vi "Initialize CVT.vi"(8 "error in (no error)":errorcluster, 11 "Measurement in":refnum<class "Measurement.lvclass">) -> (0 "error out":errorcluster, 3 "Measurement out":refnum<class "Measurement.lvclass">)   [LabVIEW 2017, in "Measurement Actor.lvlib" / "Measurement.lvclass"]
uses:
  Measurement.lvclass
  Measurement.lvclass/Measurement.ctl
  <vilib>/NI/Current Value Table/Type Defs/File Format.ctl
  <vilib>/NI/Current Value Table/Type Defs/Single Tag.ctl
  <vilib>/NI/Current Value Table/Type Defs/Data Types.ctl
  <vilib>/NI/Current Value Table/Type Defs/Tag Grouping set.ctl
  <vilib>/NI/Current Value Table/Current Value Table.lvlib
  Hardware/Hardware.lvclass
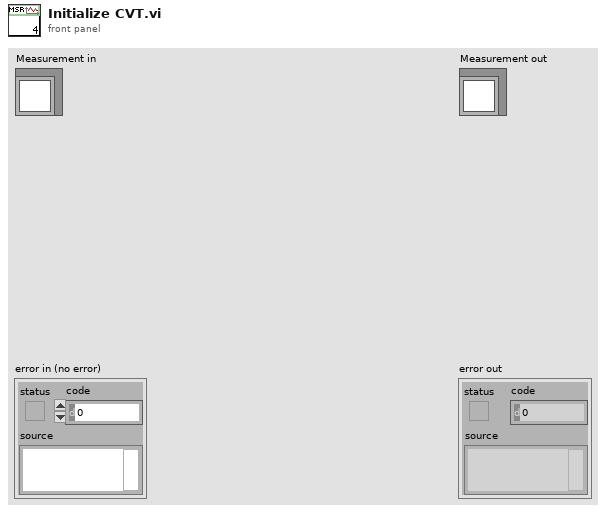
[diagram p1: front panel]
types:
  T1 = typedef "Current Value Table.lvlib/File Format.ctl" = cluster{"Tags":T2[], "Group Listings":T4[]}
  T2 = typedef "Current Value Table.lvlib/Single Tag.ctl" = cluster{"Data Type":T3, "Name":string, "Value":string, "Description":string}
  T3 = typedef "Current Value Table.lvlib/Data Types.ctl" = enum16{"Double", "Single", "I64", "I32", "I16", "I8", "U64", "U32", "U16", "U8", "String", "Boolean", "Array of U8", "Array of U16", "Array of U32", "Array of U64", "Array of I64", "Array of I32", "Array of I16", "Array of I8", "Array of Double", "Array of Single", "Array of Boolean", "Array of String"}
  T4 = typedef "Current Value Table.lvlib/Tag Grouping set.ctl" = cluster{"Group":string, "Tag Names":string[]}
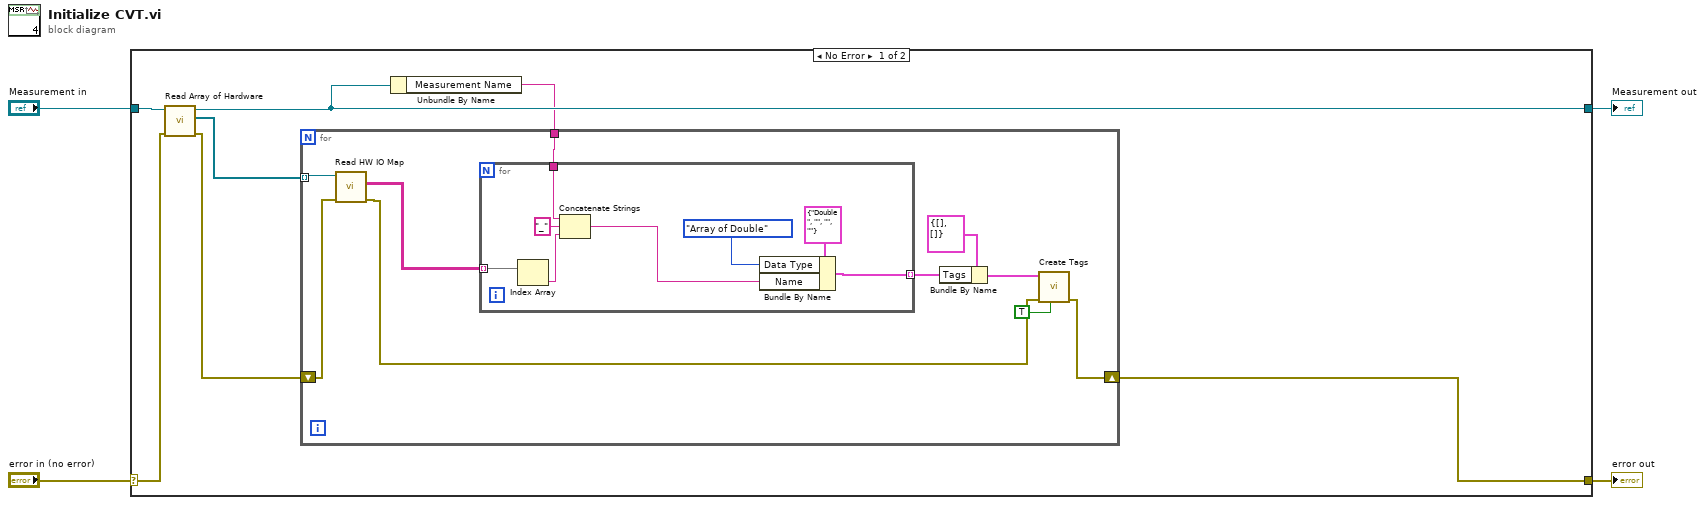
[diagram p0: block diagram]
diagram:
  n1 = case shown="No Error" "error in (no error)" {
    selector: "error in (no error)" -> [w6 w31]
    tunnel: [w5 w31] -> w3
    tunnel: [w9 w30] -> w1
    tunnel: "Measurement in" -> [w11 w30]
    frame No Error {
      n2 = call "Read Array of Hardware.vi"("error in (no error)"=w6, "Measurement in"=w11) -> ("error out"=w7:errorcluster, "Array of Hardware"=w10:refnum<class "Hardware.lvclass">[], "Measurement out"=w9:refnum<class "Measurement.lvclass">)  [unwired: 7 in]
      n3 = Unbundle By Name(w9) -> ("Measurement Name"=w8:string)
      n4 = for {
        tunnel: w10 -> [w16] mode=indexing
        tunnel: w8 -> [w18]
        shift-right: [w13] -> w5
        shift-left: w7 -> [w15]
        n5 = call "Read HW IO Map.vi"("error in (no error)"=w15, "Hardware in"=w16) -> ("error out"=w14:errorcluster, "Channel Mapping (Device -> Channel)"=w17:string[][])  [unwired: 7 in, 1 out]
        n6 = for {
          tunnel: w17 -> [w27] mode=indexing
          tunnel: [w26] -> w19 mode=indexing
          tunnel: w18 -> [w23]
          n7 = Index Array(array=w27) -> (element=w25:string)  [unwired: 1 in]
          n8 = Concatenate Strings(w23, "_" ("string"), w25) -> (w24:string)
          n9 = Bundle By Name(cluster=T2 {"Data Type"=enum."Double", "Name"="", "Value"="", "Description"=""} ("Tag"), "Data Type"=Data_Types."Array of Double", "Name"=w24) -> (w26:T2)
        }
        n10 = Bundle By Name(cluster=T1 {"Tags"=[], "Group Listings"=[]} ("CVT Tags to Create"), "Tags"=w19) -> (w21:T1)
        n11 = call <vilib>:"Create Tags.vi"("Overwrite Duplicates? (F)"=TRUE, "error in (no error)"=w14, "CVT Tags to Create"=w21) -> ("error out"=w13:errorcluster)  [unwired: 8 in]
      }
    }
    frame Error {
    }
  }
  "error out" <- w3
  "Measurement out" <- w1
